vi "State_Machine.vi"(8 "error in (no error)":errorcluster caption="entrée d'erreur (pas d'erreur)", 11 "Get_Voltage en entrée":refnum<class "Read_Weight.lvclass">) -> (0 "error out":errorcluster caption="sortie d'erreur", 2 "Json_String":string, 3 "Get_Voltage en sortie":refnum<class "Read_Weight.lvclass">)   [LabVIEW 2020, in "Library Test.lvlib" / "Read_Weight.lvclass"]
uses:
  Read_Weight.lvclass
  C:/Users/ngarcin/OneDrive - Altyor/Standard TB/Class/Test/Test (Default)/Test (Default).lvclass
  JSON API/JSON Value/Set from JSON string.vi
  Instrument/Instrument (Default)/Class Instrument (Default).lvclass
  JSON API/JSON Value/JSON Value.lvclass
  Read_Weight.lvclass/Read_Weight.ctl
  JSON API/Variant JSON/Variant JSON.lvlib
  JSON API/Get Polymorphic/JSON GetSet.lvlib
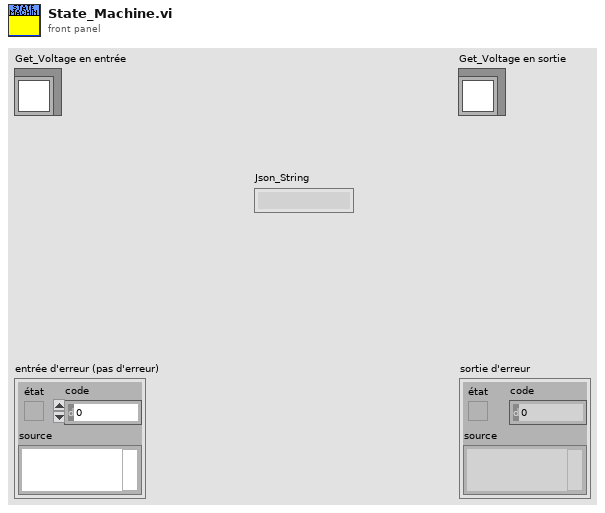
[diagram p1: front panel]
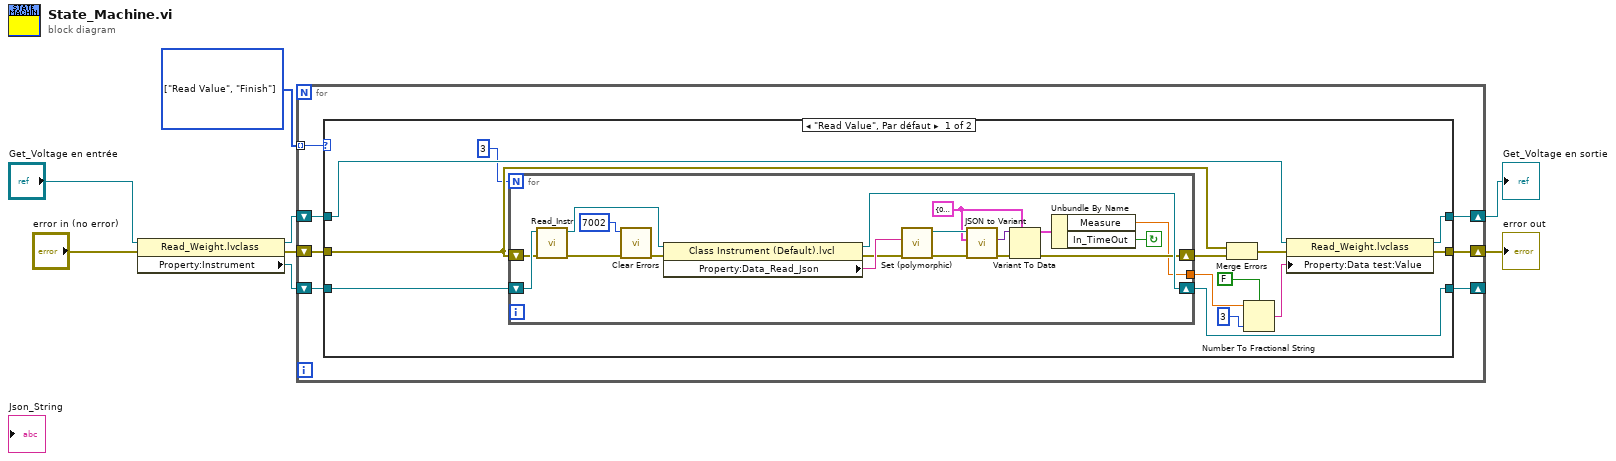
[diagram p0: block diagram]
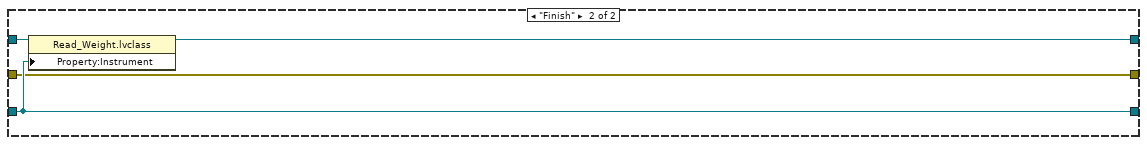
[diagram p2: hidden frame]
diagram:
  w7 = enum16{"Init", "Read Value", "Finish"}[] [enum."Read Value", enum."Finish"] items=["Init", "Read Value", "Finish"]
  n1 = property class="Read_Weight.lvclass"(reference="Get_Voltage en entrée", error in="error in (no error)") -> (reference out=w5:refnum<class "Read_Weight.lvclass">, error out=w1:errorcluster, "Property:Instrument"=w6:refnum<class "Class Instrument (Default).lvclass">)
  n2 = for {
    tunnel: w7 -> [w15] mode=indexing
    shift-right: [w13] -> _
    shift-left: w6 -> [w14]
    shift-right: [w11] -> w3
    shift-left: w5 -> [w12]
    shift-right: [w9] -> w4
    shift-left: w1 -> [w10]
    n3 = case shown="\"Read Value\", Par défaut" w15 {
      tunnel: w14 -> [w28 w48]
      tunnel: [w26 w48] -> w13
      tunnel: w12 -> [w27 w50]
      tunnel: [w24 w49] -> w11
      tunnel: w10 -> [w20 w47]
      tunnel: [w19 w47] -> w9
      frame "Read Value", Default {
        n4 = for {
          N: 3 -> [_]
          tunnel: [w33] -> w23
          shift-right: [w44] -> w26
          shift-left: w28 -> [w46]
          shift-right: [w36] -> w25
          shift-left: w20 -> [w29]
          stop <- w32 continue-if-true
          w35 = cluster{"Measure":dbl, "In_TimeOut":bool} {"Measure"=0.0, "In_TimeOut"=FALSE}
          n5 = call-dynamic "Read_Instr.vi"("error in (no error)"=w29, "Class Instrument (Default) en entrée"=w46) -> ("error out"=w43:errorcluster, "Class Instrument (Default) en sortie"=w45:refnum<class "Class Instrument (Default).lvclass">)  [unwired: 8 in]
          n6 = call <vilib>:"Clear Errors.vi"("error in (no error)"=w43, "specific error code to clear (0: all)"=7002) -> ("error out"=w31:errorcluster)  [unwired: 4 in, 1 out]
          n7 = property class="Class Instrument (Default).lvcl"(reference=w45, error in=w31) -> (reference out=w44:refnum<class "Class Instrument (Default).lvclass">, error out=w38:errorcluster, "Property:Data_Read_Json"=w39:string)
          n8 = call-poly "Set (polymorphic).vi"("error in (no error)"=w38, "JSON stream"=w39) -> ("error out"=w42:errorcluster, "JSON Value out"=w40:refnum<class "JSON Value.lvclass">)  [unwired: 7 in, 1 out]
          n9 = call "JSON to Variant.vi"("error in (no error)"=w42, "Variant (Data Type)"=w35, "JSON Value"=w40) -> ("error out"=w41:errorcluster, "Variant out"=w37:variant)  [unwired: 7 in]
          n10 = Variant To Data(error in=w41, type=w35, Variant=w37) -> (data=w34:cluster{"Measure":dbl, "In_TimeOut":bool}, error out=w36:errorcluster)
          n11 = Unbundle By Name(w34) -> ("Measure"=w33:dbl, "In_TimeOut"=w32:bool)
        }
        n12 = Merge Errors(w20, w25) -> (w21:errorcluster)
        n13 = Number To Fractional String(use system decimal point (T)=FALSE ("utiliser le séparateur décimal du système (V)"), number=w23, precision (6)=i16 3 ("précision (6)")) -> (F-format string=w22:string)  [unwired: 1 in]
        n14 = property class="Read_Weight.lvclass"(reference=w27, error in=w21, "Property:Data test:Value"=w22) -> (reference out=w24:refnum<class "Read_Weight.lvclass">, error out=w19:errorcluster)
      }
      frame "Finish" {
        n15 = property class="Read_Weight.lvclass"(reference=w50, "Property:Instrument"=w48) -> (reference out=w49:refnum<class "Read_Weight.lvclass">)  [unwired: 1 in, 1 out]
      }
    }
  }
  "error out" <- w4
  "Get_Voltage en sortie" <- w3
